vi "GOOP_VirtualFolder_Item_OnPopUpMenu.vi"(11 "Object":u64) -> ()   [LabVIEW 2020]
uses:
  <resource>/Framework/Providers/API/mxLvMenuItem.ctl
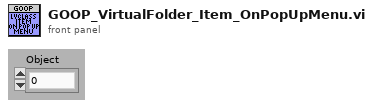
[diagram p1: front panel]
types:
  T1 = typedef "mxLvMenuItem.ctl" = cluster{"Menu Name":string, "Description":string, "Icon File Name":path, "Menu Tag":string, "Enabled":bool, "Checked":bool, "Separator":bool, "Batchable":bool, "Weight":i32, "Batch Mode (Ignored if Not Batchable)":enum32{"Show If All Items Support Command", "Show If Any Items Support Command"}, "Menu Location":enum32{"<None>", "Project", "Project / Build Specifications", "Tools", "Tools / Source Control", "Tools / Real-Time Module", "Help"}, "Exclude From Getting Started Window Menu":bool}
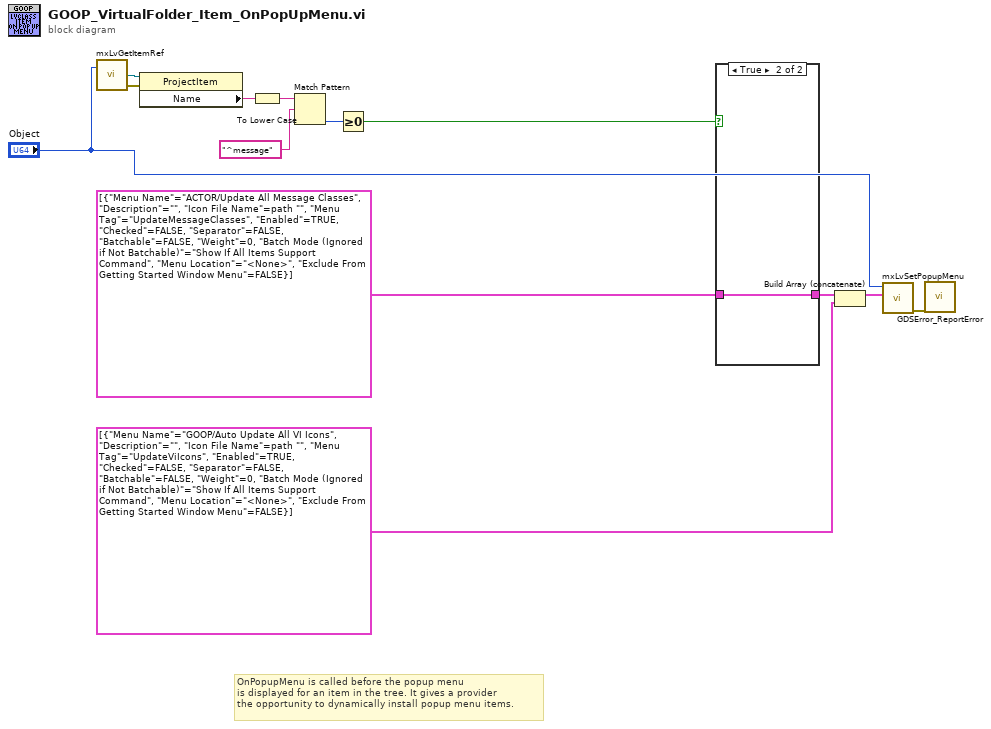
[diagram p0: block diagram]
diagram:
  # "OnPopupMenu is called before the popup menu\nis displayed for an item in the tree. It gives a provider\nthe opportunity to dynamically install popup menu items."
  n1 = call <resource>:"mxLvGetItemRef.vi"("Item"="Object") -> ("Item Refnum"=w9:refnum<vi>, "error out"=w7:errorcluster)  [unwired: 1 in, 1 out]
  n2 = property class="ProjectItem"(reference=w9, error in=w7) -> ("Name"=w11:string)  [unwired: 2 out]
  n3 = To Lower Case(string=w11) -> (all lower case string=w12:string)
  n4 = Match Pattern(string=w12, regular expression="^message") -> (offset past match=w10:i32)  [unwired: 1 in, 3 out]
  n5 = Greater Or Equal To 0?(x=w10) -> (x >= 0?=w6:bool)
  n6 = case shown="True" w6 {
    tunnel: T1[] [{"Menu Name"="ACTOR/Update All Message Classes", "Description"="", "Icon File Name"=path "", "Menu Tag"="UpdateMessageClasses", "Enabled"=TRUE, "Checked"=FALSE, "Separator"=FALSE, "Batchable"=FALSE, "Weight"=0, "Batch Mode (Ignored if Not Batchable)"=enum."Show If All Items Support Command", "Menu Location"=enum."<None>", "Exclude From Getting Started Window Menu"=FALSE}] -> [_ w14]
    tunnel: [_ w14] -> w3
    frame False {
    }
    frame True {
    }
  }
  n7 = Build Array (concatenate)(w3, T1[] [{"Menu Name"="GOOP/Auto Update All VI Icons", "Description"="", "Icon File Name"=path "", "Menu Tag"="UpdateViIcons", "Enabled"=TRUE, "Checked"=FALSE, "Separator"=FALSE, "Batchable"=FALSE, "Weight"=0, "Batch Mode (Ignored if Not Batchable)"=enum."Show If All Items Support Command", "Menu Location"=enum."<None>", "Exclude From Getting Started Window Menu"=FALSE}]) -> (w1:T1[])
  n8 = call <resource>:"mxLvSetPopupMenu.vi"("Popup Menu Items"=w1, "Item"="Object") -> ("error out"=w5:errorcluster)  [unwired: 8 in, 1 out]
  n9 = call "GDSError_ReportError.vi"("error in (no error)"=w5) -> ()  [unwired: 18 in, 1 out]
